vi "FanPressure2.vi"() -> ()   [LabVIEW 2024]
uses:
  <vilib>/drjdpowell/SQLite Library/SQL Connection/Connection.lvclass
  <vilib>/Instr/_visa.llb/VISA Find Search Mode.ctl
  <vilib>/drjdpowell/SQLite Library/SQL Connection/Open (path).vi
  <vilib>/Analysis/baseanly.llb/Mean (DBL).vi
  <vilib>/drjdpowell/SQLite Library/SQL Connection/Open (string).vi
  <vilib>/Instr/_visa.llb/VISA Configure Serial Port (Instr).vi
  <vilib>/drjdpowell/SQLite Library/SQL Connection/Execute SQL (No results).vi
  <vilib>/AdvancedString/Path To Command Line String.vi
  <vilib>/Analysis/NI_AALBase.lvlib
  <vilib>/drjdpowell/SQLite Library/SQLite.lvlib
panel:
  out "Array":string[](array[string])
  in  "Pause":bool
  out "DC Power":bool
  in  "Message":string
  out "Receive Type":T1
  out "user event out":refnum<user-event>
  out "Table Name":string
  out "Table Created":bool
  out "time string":string
  out "date string":string
  out "SQLite Connection":refnum<class "Connection.lvclass">
  in  "View Data":bool
  in  "Reset Plot":bool
  in  "Write To Database":bool
  in  "Interval Time":u32=200
  out "Fan Speed":i32
  out "Fan Shunt Voltage":u16
  out "Fan Power":sgl
  out "Fan current":sgl
  out "Fan Voltage":sgl
  in  "Speed Control":enum32{"Values", "Paramters"}(tab)
  in  "Control Mode":enum32{"Auto", "Manual"}(radio)=enum."Manual"
  in  "Speed Setup":u16=2000 min=10 max=36 step=1
  in  "Output":sgl(knob) min=0 max=12 step=0.1 scale=0.0..12.0 scale format="%.1f"
  in  "Min Voltage":u32 max=12 step=1
  in  "Max Voltage":u32=12 min=12 max=36
  in  "Parameter Read Button":bool
  in  "Parameter Write Button":bool
  in  "Fan Speed At Full Output":u32
  in  "Fan Speed At 50% Output":u32
  in  "KD":sgl
  in  "KI":sgl=0.0002
  in  "KP":sgl=0.008
  in  "Write Data":bool
  in  "Start Button":bool
  out "MCU":bool
  out "Serial Port":refnum<visa-resource-name>
  in  "stop":bool
  in  "Tab Control":enum32{"Readings", "Raw Data"}(tab)
  out "Waveform Chart 2":dbl[][](graph)
  out "Waveform Chart":sgl[][](graph)
  out "data":dynamicdata(graph) caption="Raw Data"
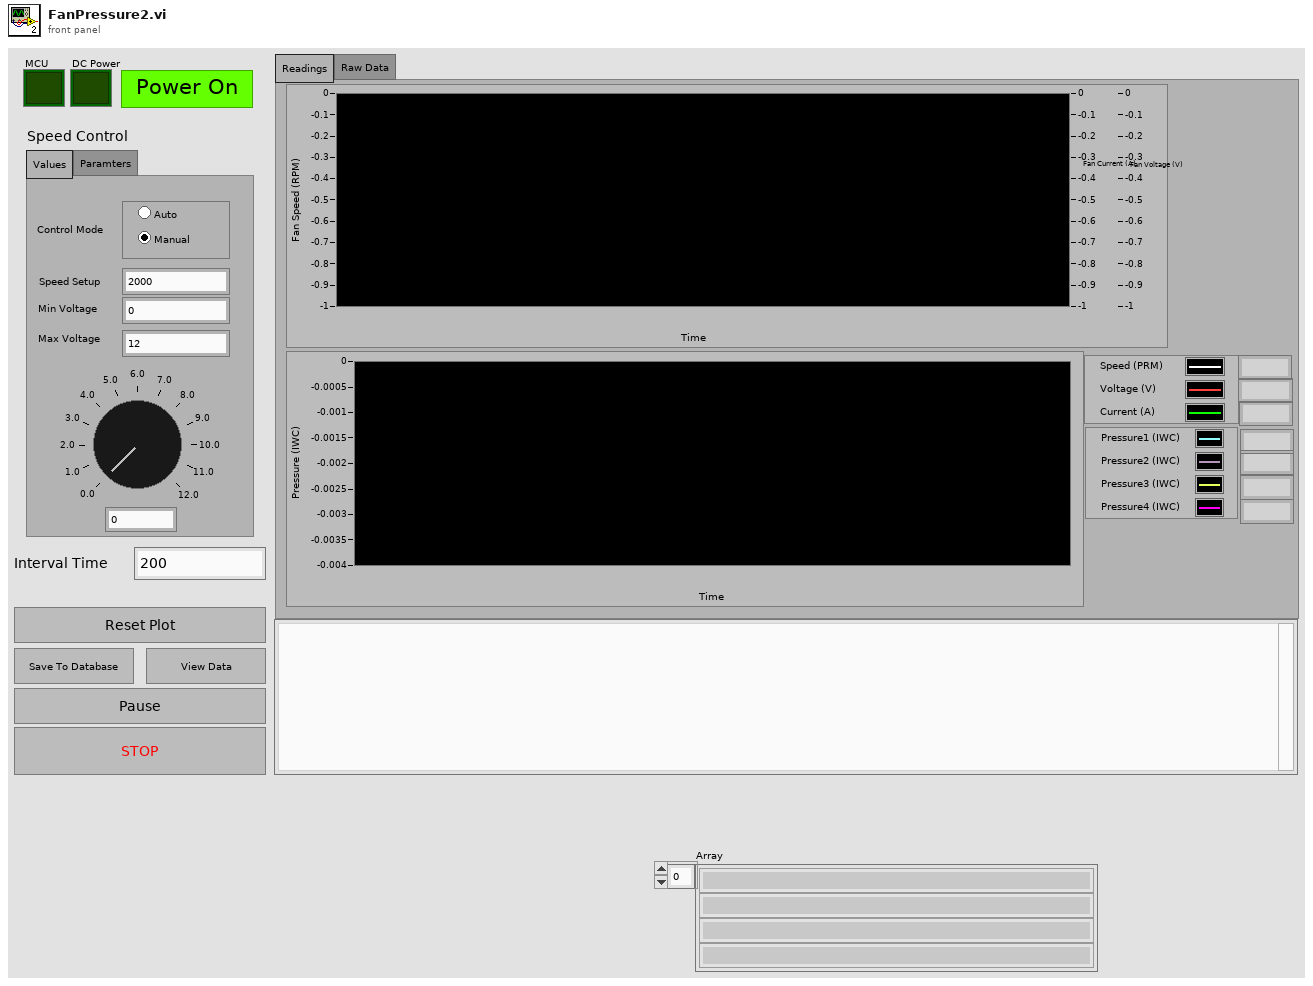
[diagram p1: front panel]
types:
  T1 = cluster{u8, u8, u8, u8, u16, u16, i16, i16, i16, i16, u16, u16, u16, u16, u16, u16, sgl, sgl, sgl, u32, u32, u8, u8, u8, u8}
  T2 = enum16{"New or existing", "Existing", "Read only"}
  T3 = enum8{"Enabled", "Disabled", "Disabled and Grayed Out"}
  T4 = enum32{"Invalid", "Standard", "Closed", "Hidden", "Minimized", "Maximized"}
  T5 = cluster{u32, "Fan current":sgl, "Fan current":sgl, "Fan current":sgl, "Fan Power":sgl, sgl, sgl, sgl, sgl, sgl, "Output":sgl, "Output":sgl}
  T6 = enum16{"big-endian, network order", "native, host order", "little-endian"}
  T7 = typedef "VISA Find Search Mode.ctl" = u32
  T8 = cluster{"y":u8, "y":u8, "y":u8, u8, u16, "Speed Setup":u16, u16, u16, "y":u8, "y":u8, "y":u8, "y":u8}
  T9 = cluster{"y":u8, "y":u8, "y":u8, "y":u8, "KP":sgl, "KI":sgl, "KD":sgl, "Fan Speed At 50% Output":u32, "Fan Speed At Full Output":u32, "y":u8, "y":u8, "y":u8, "y":u8}
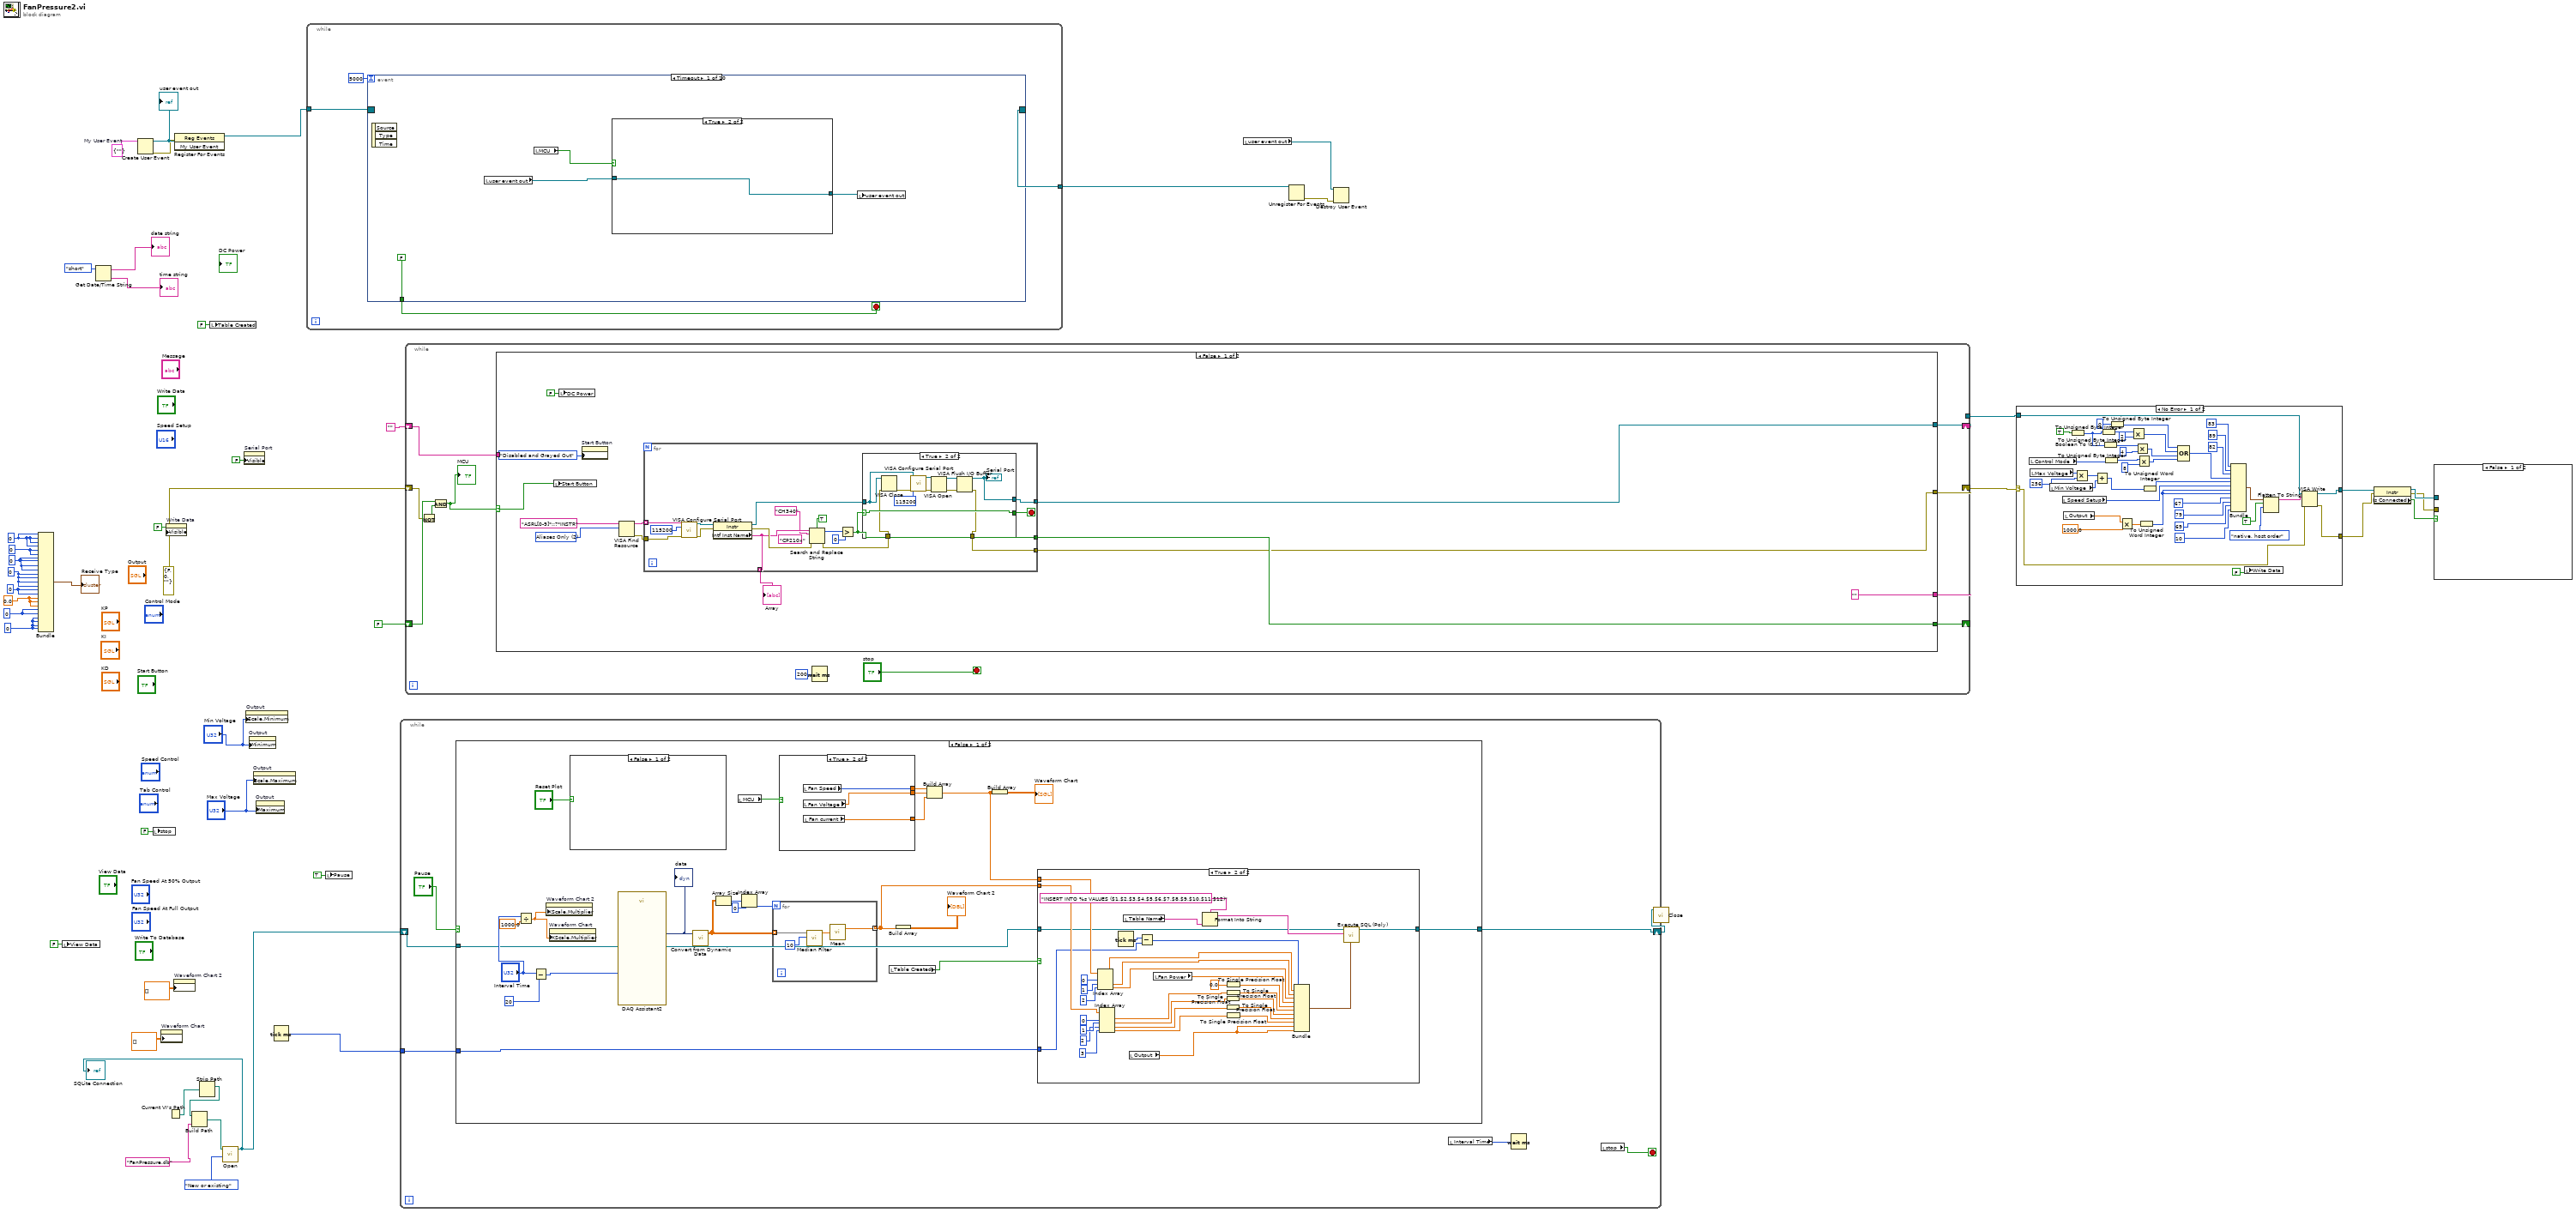
[diagram p0: block diagram]
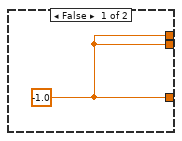
[diagram p3: hidden frame]
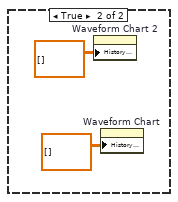
[diagram p4: hidden frame]
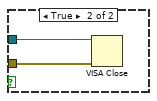
[diagram p6: hidden frame]
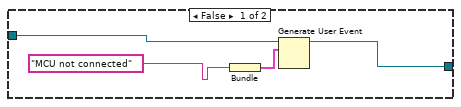
[diagram p8: hidden frame]
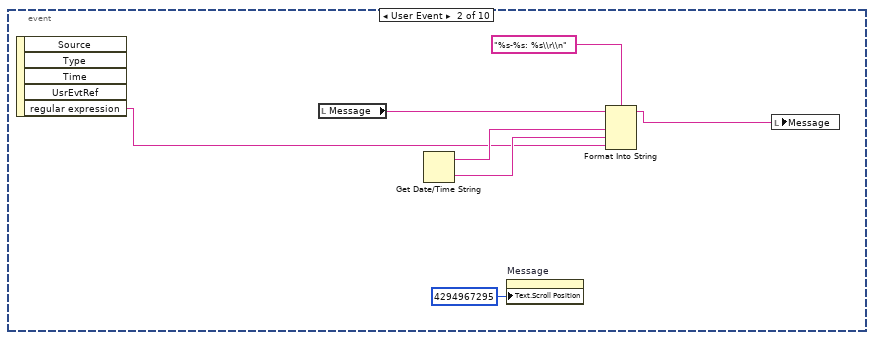
[diagram p9: hidden frame]
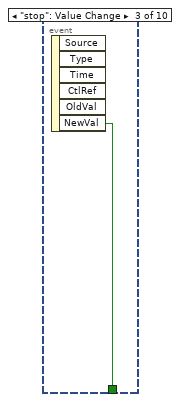
[diagram p10: hidden frame]
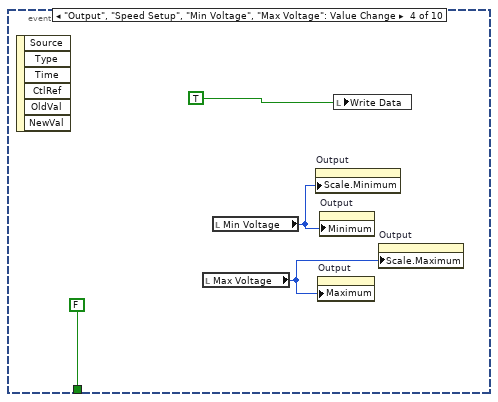
[diagram p11: hidden frame]
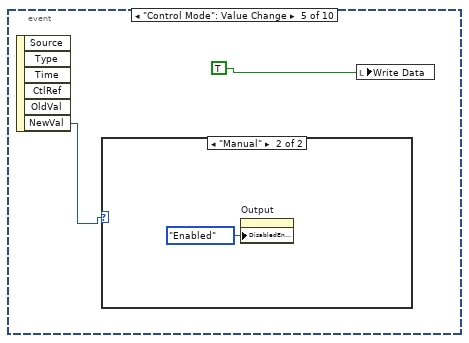
[diagram p12: hidden frame]
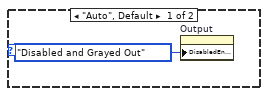
[diagram p13: hidden frame]
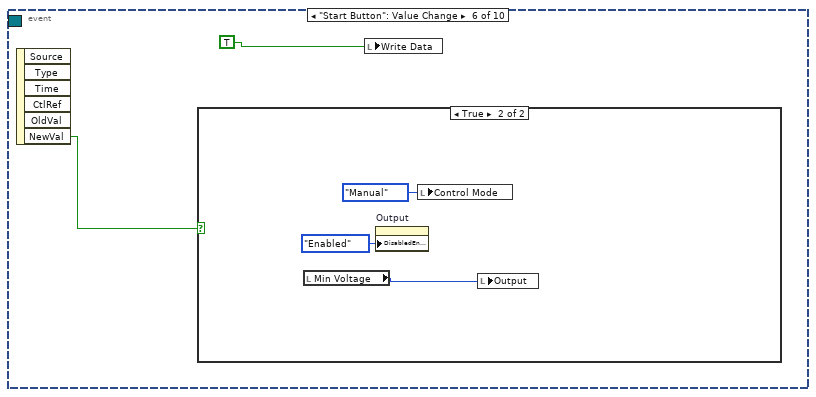
[diagram p14: hidden frame]
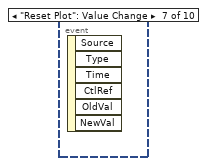
[diagram p16: hidden frame]
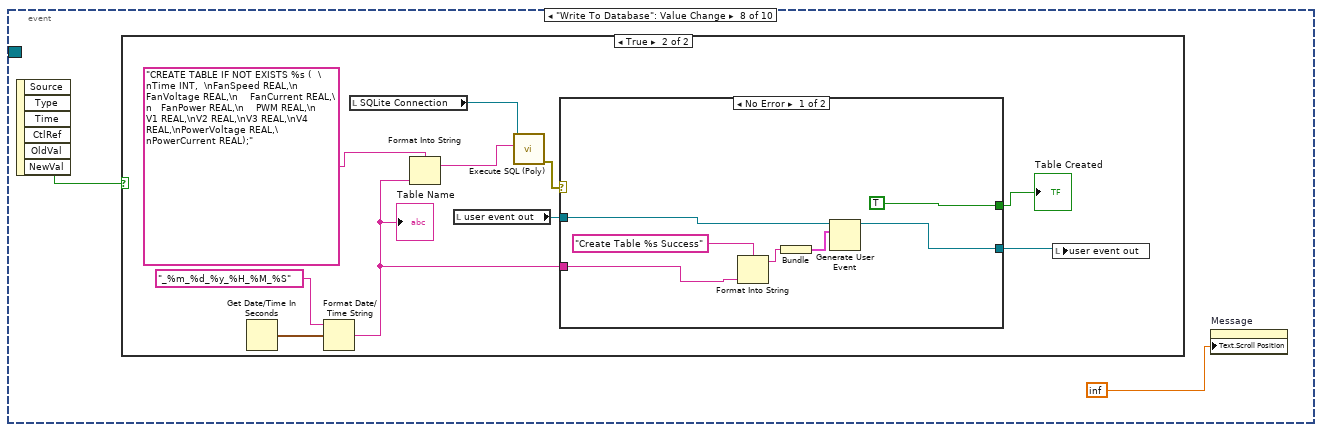
[diagram p17: hidden frame]
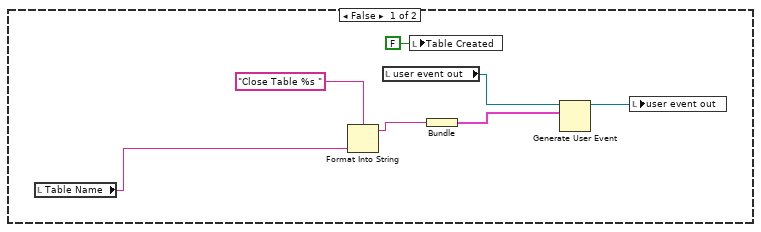
[diagram p18: hidden frame]
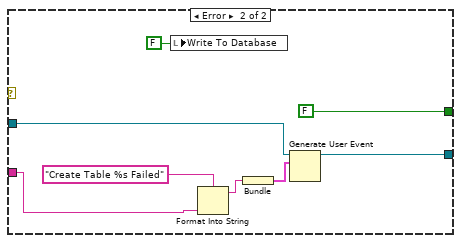
[diagram p19: hidden frame]
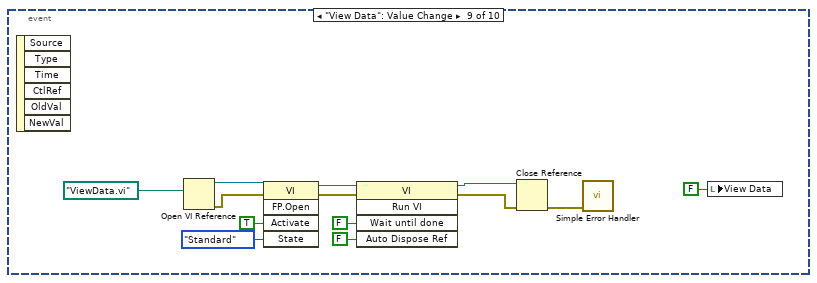
[diagram p20: hidden frame]
diagram:
  w3 = u32 0
  w4 = sgl 0.0
  w23 = cluster{"regular expression":string} {"regular expression"=""}  # My User Event
  w39 = u16 0
  w5 = u8 0
  w41 = i16 0
  w40 = u16 0
  w42 = u16 0
  w43 = u8 0
  n1 = Bundle(w43, w43, w43, w43, w42, w42, w41, w41, w41, w41, w39, w39, w39, w39, w40, w40, w4, w4, w4, w3, w3, w5, w5, w5, w5) -> (→"Receive Type":T1)  [unwired: 1 in]
  n2 = local write "View Data"(FALSE ("View Data")) -> ()
  n3 = Get Date/Time String(date format (0)=enum16{"short", "long", "abbreviated"}."short") -> (date string=→"date string":string, time string=→"time string":string)  [unwired: 2 in]
  n4 = Create User Event(user event datatype=w23) -> (user event=w22:refnum<user-event>, error out=w20:errorcluster)  [unwired: 1 in]
  "user event out" <- w22
  n5 = local write "stop"(FALSE ("stop")) -> ()
  n6 = property on="Waveform Chart" class="WFChart (strict)"("History Data"=dbl[][] []) -> ()  [unwired: 2 in, 2 out]
  n7 = property on="Write Data" class="Bool (strict)"("Visible"=FALSE) -> ()  [unwired: 2 in, 2 out]
  n8 = Current VI's Path() -> (path=w14:path)
  n9 = property on="Waveform Chart 2" class="WFChart (strict)"("History Data"=dbl[][] []) -> ()  [unwired: 2 in, 2 out]
  n10 = register-events(error in=w20, w22) -> (reference out=w21:refnum<event-registration>)  [unwired: 1 in, 1 out]
  n11 = Strip Path(path=w14) -> (stripped path=w13:path)  [unwired: 1 out]
  n12 = Build Path(base path=w13, name or relative path="FanPressure.db" ("db file")) -> (appended path=w15:path)
  n13 = local write "Table Created"(FALSE ("Table Created")) -> ()
  n14 = call-poly <vilib>:"Open.vi"("File Option"=T2."New or existing", "db file"=w15) -> ("SQLite Connection"=w12:refnum<class "Connection.lvclass">)  [unwired: 8 in, 1 out]
  "SQLite Connection" <- w12
  n15 = property on="Serial Port" class="VISAName"("Visible"=FALSE) -> ()  [unwired: 2 in, 2 out]
  n16 = property on="Output" class="Knob (strict)"("Scale.Minimum"="Min Voltage") -> ()  [unwired: 2 in, 2 out]
  n17 = property on="Output" class="Knob (strict)"("Minimum"="Min Voltage") -> ()  [unwired: 2 in, 2 out]
  n18 = property on="Output" class="Knob (strict)"("Scale.Maximum"="Max Voltage") -> ()  [unwired: 2 in, 2 out]
  n19 = property on="Output" class="Knob (strict)"("Maximum"="Max Voltage") -> ()  [unwired: 2 in, 2 out]
  n20 = Tick Count (ms)() -> (millisecond timer value=w9:u32)
  n21 = while {
    tunnel: w21 -> [w50]
    tunnel: [w49] -> w19
    stop <- w51 stop-if-true
    n22 = event shown="[0] Timeout" {
      selector: w50 -> [_ _ _ _ _ _ _ _ _ _]
      dyn-events: [_ _ _ _ _ _ _ _ _ _] -> w49
      timeout: 5000 -> [_ _ _ _ _ _ _ _ _ _]
      tunnel: [FALSE ("NewVal") _ w68 FALSE ("NewVal") _ _ _ _ _ _] -> w51
      event Timeout {
        n23 = event-data() -> ()  [unwired: 1 in, 3 out]
        n24 = local read "user event out"() -> (w54:refnum<user-event>)
        n25 = local read "MCU"() -> (w52:bool)
        n26 = case shown="True" w52 {
          tunnel: w54 -> [w57 w60]
          tunnel: [w58 w60] -> w53
          frame False {
            n27 = Bundle("format string"="MCU not connected") -> (w59:cluster{"format string":string})  [unwired: 1 in]
            n28 = Generate User Event(user event=w57, event data cluster=w59) -> (user event out=w58:refnum<user-event>)  [unwired: 2 in, 1 out]
          }
          frame True {
          }
        }
        n29 = local write "user event out"(w53) -> ()
      }
      event User Event {
        n30 = event-data() -> ("regular expression"=w62:string)  [unwired: 1 in, 4 out]
        n31 = local read "Message"() -> (w67:string)
        n32 = Get Date/Time String() -> (date string=w66:string, time string=w65:string)  [unwired: 3 in]
        n33 = property on="Message" class="Str"("Text.Scroll Position"=u32 4294967295) -> ()  [unwired: 2 in, 2 out]
        n34 = Format Into String(format string="%s-%s: %s\\r\\n", initial string=w67, w66, w65, w62) -> (resulting string=w64:string)  [unwired: 1 in, 1 out]
        n35 = local write "Message"(w64) -> ()
      }
      event "stop": Value Change {
        n36 = event-data() -> ("NewVal"=w68:bool)  [unwired: 1 in, 5 out]
      }
      event "Output", "Speed Setup", "Min Voltage", "Max Voltage": Value Change {
        n37 = event-data() -> ()  [unwired: 1 in, 6 out]
        n38 = local read "Max Voltage"() -> (w69:u32)
        n39 = local read "Min Voltage"() -> (w70:u32)
        n40 = property on="Output" class="Knob (strict)"("Scale.Minimum"=w70) -> ()  [unwired: 2 in, 2 out]
        n41 = property on="Output" class="Knob (strict)"("Maximum"=w69) -> ()  [unwired: 2 in, 2 out]
        n42 = property on="Output" class="Knob (strict)"("Minimum"=w70) -> ()  [unwired: 2 in, 2 out]
        n43 = local write "Write Data"(TRUE ("Write Data")) -> ()
        n44 = property on="Output" class="Knob (strict)"("Scale.Maximum"=w69) -> ()  [unwired: 2 in, 2 out]
      }
      event "Control Mode": Value Change {
        n45 = event-data() -> ("NewVal"=w73:enum32{"Auto", "Manual"})  [unwired: 1 in, 5 out]
        n46 = case shown="\"Manual\"" w73 {
          frame "Auto", Default {
            n47 = property on="Output" class="Knob (strict)"("DisabledEnum"=T3."Disabled and Grayed Out" ("Disabled")) -> ()  [unwired: 2 in, 2 out]
          }
          frame "Manual" {
            n48 = property on="Output" class="Knob (strict)"("DisabledEnum"=T3."Enabled" ("Disabled")) -> ()  [unwired: 2 in, 2 out]
          }
        }
        n49 = local write "Write Data"(TRUE ("Write Data")) -> ()
      }
      event "Start Button": Value Change {
        n50 = event-data() -> ("NewVal"=w77:bool)  [unwired: 1 in, 5 out]
        n51 = case shown="True" w77 {
          frame False {
          }
          frame True {
            n52 = local read "Min Voltage"() -> (w80:u32)
            n53 = property on="Output" class="Knob (strict)"("DisabledEnum"=T3."Enabled" ("Disabled")) -> ()  [unwired: 2 in, 2 out]
            n54 = local write "Control Mode"(enum32{"Auto", "Manual"}."Manual" ("Control Mode")) -> ()
            n55 = local write "Output"(w80) -> ()
          }
        }
        n56 = local write "Write Data"(TRUE ("Write Data")) -> ()
      }
      event "Reset Plot": Value Change {
        n57 = event-data() -> ()  [unwired: 1 in, 6 out]
      }
      event "Write To Database": Value Change {
        n58 = event-data() -> ("NewVal"=w83:bool)  [unwired: 1 in, 5 out]
        n59 = case shown="True" w83 {
          frame False {
            n60 = local read "Table Name"() -> (w89:string)
            n61 = Format Into String(format string="Close Table %s ", w89) -> (resulting string=w86:string)  [unwired: 2 in, 1 out]
            n62 = local read "user event out"() -> (w87:refnum<user-event>)
            n63 = local write "Table Created"(FALSE ("Table Created")) -> ()
            n64 = Bundle(w86) -> (w85:cluster{string})  [unwired: 1 in]
            n65 = Generate User Event(user event=w87, event data cluster=w85) -> (user event out=w84:refnum<user-event>)  [unwired: 2 in, 1 out]
            n66 = local write "user event out"(w84) -> ()
          }
          frame True {
            n67 = Get Date/Time In Seconds() -> (seconds since 1Jan1904=w99:timestamp)
            n68 = Format Date/Time String(time format string (%c)="_%m_%d_%y_%H_%M_%S", seconds (now)=w99) -> (date/time string=w91:string)  [unwired: 1 in]
            "Table Name" <- w91
            n69 = local read "SQLite Connection"() -> (w100:refnum<class "Connection.lvclass">)
            n70 = Format Into String(format string="CREATE TABLE IF NOT EXISTS %s (  \nTime INT,  \nFanSpeed REAL,\n    FanVoltage REAL,\n    FanCurrent REAL,\n   FanPower REAL,\n    PWM REAL,\n    V1 REAL,\nV2 REAL,\nV3 REAL,\nV4 REAL,\nPowerVoltage REAL,\nPowerCurrent REAL);" ("SQL"), w91) -> (resulting string=w96:string)  [unwired: 2 in, 1 out]
            n71 = local read "user event out"() -> (w93:refnum<user-event>)
            n72 = call-poly <vilib>:"Execute SQL (Poly).vi"("SQL"=w96, "SQLite Connection in"=w100) -> ("error out"=w95:errorcluster)  [unwired: 8 in, 1 out]
            n73 = case shown="No Error" w95 {
              tunnel: [TRUE ("Table Created") FALSE ("Table Created")] -> w94
              tunnel: w93 -> [w101 w110]
              tunnel: [w102 w109] -> w92
              tunnel: w91 -> [w103 w108]
              frame No Error {
                n74 = Format Into String(format string="Create Table %s Success", w103) -> (resulting string=w106:string)  [unwired: 2 in, 1 out]
                n75 = Bundle(w106) -> (w105:cluster{string})  [unwired: 1 in]
                n76 = Generate User Event(user event=w101, event data cluster=w105) -> (user event out=w102:refnum<user-event>)  [unwired: 2 in, 1 out]
              }
              frame Error {
                n77 = local write "Write To Database"(FALSE ("Write To Database")) -> ()
                n78 = Format Into String(format string="Create Table %s Failed", w108) -> (resulting string=w113:string)  [unwired: 2 in, 1 out]
                n79 = Bundle(w113) -> (w112:cluster{string})  [unwired: 1 in]
                n80 = Generate User Event(user event=w110, event data cluster=w112) -> (user event out=w109:refnum<user-event>)  [unwired: 2 in, 1 out]
              }
            }
            "Table Created" <- w94
            n81 = local write "user event out"(w92) -> ()
          }
        }
        n82 = property on="Message" class="Str"("Text.Scroll Position"=inf) -> ()  [unwired: 2 in, 2 out]
      }
      event "View Data": Value Change {
        n83 = event-data() -> ()  [unwired: 1 in, 6 out]
        n84 = Open VI Reference(vi path=path "ViewData.vi") -> (vi reference=w126:refnum<vi>, error out=w119:errorcluster)  [unwired: 5 in]
        n85 = invoke class="VI" method="FP.Open"(reference=w126, error in=w119, "Activate"=TRUE ("Activate?"), "State"=T4."Standard") -> (reference out=w123:refnum<vi>, error out=w122:errorcluster)  [unwired: 1 in, 3 out]
        n86 = invoke class="VI" method="Run VI"(reference=w123, error in=w122, "Wait until done"=FALSE ("Wait Until Done"), "Auto Dispose Ref"=FALSE ("Auto Dispose Reference")) -> (reference out=w118:refnum<vi>, error out=w117:errorcluster)  [unwired: 1 in, 3 out]
        n87 = Close Reference(reference=w118, error in (no error)=w117) -> (error out=w116:errorcluster)
        n88 = call <vilib>:"Simple Error Handler.vi"("error in (no error)"=w116) -> ()  [unwired: 4 in, 5 out]
        n89 = local write "View Data"(FALSE ("View Data")) -> ()
      }
      event "Message": Value Change {
        n90 = event-data() -> ()  [unwired: 1 in, 6 out]
      }
    }
  }
  n91 = local write "Pause"(TRUE ("Pause")) -> ()
  n92 = while {
    shift-right: [w132] -> w11
    shift-left: w12 -> [w131]
    tunnel: w9 -> [w130]
    stop <- w134 stop-if-true
    n93 = case shown="False" "Pause" {
      tunnel: [w137 w202] -> w132
      tunnel: w131 -> [w136 w202]
      tunnel: w130 -> [w135 _]
      frame False {
        n94 = Divide(x="Interval Time", y=1000.0) -> (x/y=w146:dbl)
        n95 = Subtract(x="Interval Time", y=u32 20) -> (x-y=w155:u32)
        n96 = property on="Waveform Chart 2" class="WFChart (strict)"("XScale.Multiplier"=w146) -> ()  [unwired: 2 in, 2 out]
        n97 = property on="Waveform Chart" class="WFChart (strict)"("XScale.Multiplier"=w146) -> ()  [unwired: 2 in, 2 out]
        n98 = case shown="False" "Reset Plot" {
          frame False {
          }
          frame True {
            n99 = property on="Waveform Chart 2" class="WFChart (strict)"("History Data"=dbl[][] []) -> ()  [unwired: 2 in, 2 out]
            n100 = property on="Waveform Chart" class="WFChart (strict)"("History Data"=dbl[][] []) -> ()  [unwired: 2 in, 2 out]
          }
        }
        n101 = call "DAQ Assistant2"("number of samples"=w155) -> ("data"=w157:dynamicdata)  [unwired: 16 in, 2 out]
        "data" <- w157
        n102 = call "Convert from Dynamic Data"("Dynamic Data Type"=w157) -> ("Array"=w154:dbl[][])  [unwired: 3 in]
        n103 = Array Size(array=w154) -> (size(s)=w153:i32[])
        n104 = local read "MCU"() -> (w145:bool)
        n105 = Index Array(array=w153, index=0) -> (element=w151:i32)
        n106 = for {
          N: w151 -> [_]
          tunnel: w154 -> [w201] mode=indexing
          tunnel: [w198] -> w140 mode=indexing
          n107 = call <vilib>:"Median Filter.vi"("left rank"=10, "X"=w201) -> ("Filtered X"=w199:dbl[])  [unwired: 8 in, 1 out]
          n108 = call-poly <vilib>:"Mean.vi"("X"=w199) -> ("mean"=w198:dbl)  [unwired: 1 out]
        }
        n109 = case shown="True" w145 {
          tunnel: [w192 w195] -> w144
          tunnel: [w192 w194] -> w143
          tunnel: [w192 w193] -> w142
          frame False {
            w192 = sgl -1.0 ("Fan current")
          }
          frame True {
            n110 = local read "Fan Speed"() -> (w193:i32)
            n111 = local read "Fan Voltage"() -> (w194:sgl)
            n112 = local read "Fan current"() -> (w195:sgl)
          }
        }
        n113 = local read "Table Created"() -> (w138:bool)
        n114 = Build Array(w140) -> (→"Waveform Chart 2":dbl[][])
        n115 = Build Array(w142, w143, w144) -> (w139:sgl[])
        n116 = Build Array(w139) -> (→"Waveform Chart":sgl[][])
        n117 = case shown="True" w138 {
          tunnel: w140 -> [_ w187]
          tunnel: w139 -> [_ w191]
          tunnel: w136 -> [w158 w174]
          tunnel: [w158 w173] -> w137
          tunnel: w135 -> [_ w162]
          frame False {
          }
          frame True {
            n118 = Index Array(array=w191, index #1=0 ("index"), index #2=1 ("index"), index #3=2 ("index")) -> (element #1=w182:sgl, element #2=w181:sgl, element #3=w180:sgl)
            n119 = Index Array(array=w187, index #1=0 ("index"), index #2=1 ("index"), index #3=2 ("index"), index #4=3 ("index")) -> (element #1=w166:dbl, element #2=w168:dbl, element #3=w170:dbl, element #4=w172:dbl)
            n120 = Tick Count (ms)() -> (millisecond timer value=w163:u32)
            n121 = local read "Table Name"() -> (w176:string)
            n122 = local read "Output"() -> (w159:sgl)
            n123 = Subtract(x=w163, y=w162) -> (x-y=w161:u32)
            n124 = local read "Fan Power"() -> (w179:sgl)
            n125 = Format Into String(format string="INSERT INTO %s VALUES ($1,$2,$3,$4,$5,$6,$7,$8,$9,$10,$11,$12)" ("SQL"), w176) -> (resulting string=w175:string)  [unwired: 2 in, 1 out]
            n126 = To Single Precision Float(number=w168) -> (single precision float=w167:sgl)
            n127 = To Single Precision Float(number=w170) -> (single precision float=w169:sgl)
            n128 = To Single Precision Float(number=sgl 0.0) -> (single precision float=w164:sgl)
            n129 = To Single Precision Float(number=w166) -> (single precision float=w165:sgl)
            n130 = To Single Precision Float(number=w172) -> (single precision float=w171:sgl)
            n131 = Bundle(w161, "Fan current"=w182, "Fan current"=w181, "Fan current"=w180, "Fan Power"=w179, w164, w165, w167, w169, w171, "Output"=w159, "Output"=w159) -> (w178:T5)  [unwired: 1 in]
            n132 = call-poly <vilib>:"Execute SQL (Poly).vi"("Parameter(s)"=w178, "SQL"=w175, "SQLite Connection in"=w174) -> ("SQLite Connection"=w173:refnum<class "Connection.lvclass">)  [unwired: 7 in, 1 out]
          }
        }
      }
      frame True {
      }
    }
    n133 = local read "Interval Time"() -> (w133:u32)
    n134 = Wait (ms)(milliseconds to wait=w133) -> ()  [unwired: 1 out]
    n135 = local read "stop"() -> (w134:bool)
  }
  n136 = while {
    shift-right: [w212] -> _
    shift-left: FALSE -> [w210]
    shift-right: [w211] -> w36
    shift-left: errorcluster {"status"=FALSE, "code"=0, "source"=""} ("error in (no error)") -> [w206]
    tunnel: [w208] -> w37
    shift-right: [w205] -> _
    shift-left: "" -> [w204]
    stop <- "stop" stop-if-true
    n137 = Not(x=w206) -> (.not. x?=w209:bool)
    n138 = And(x=w210, y=w209) -> (x .and. y?=w203:bool)
    "MCU" <- w203
    n139 = case shown="False" w203 {
      selector: w203 -> [w217 w271]
      tunnel: [w221 w271] -> w212
      tunnel: [w220 w264] -> w211
      tunnel: [w219 w266] -> w208
      tunnel: w204 -> [_ w276]
      tunnel: ["" w260] -> w205
      frame False {
        w224 = T7 2 items=["Canonical Names Only"=0, "Aliases Only"=2, "Include Matching Aliases"=3, "Include All Aliases"=4] ("Search Mode")
        n140 = local write "Start Button"(w217) -> ()
        n141 = local write "DC Power"(FALSE ("DC Power")) -> ()
        n142 = property on="Start Button" class="Bool (strict)"("DisabledEnum"=T3."Disabled and Grayed Out" ("Disabled")) -> ()  [unwired: 2 in, 2 out]
        n143 = VISA Find Resource(10:w224, 11:"ASRL[0-9]*::?*INSTR" ("expression (\"?*\")")) -> (0:w222:errorcluster, 3:w223:string[])  [unwired: 1 in, 1 out]
        n144 = for {
          tunnel: w223 -> [w232] mode=indexing
          tunnel: w222 -> [w242]
          tunnel: [w236] -> w221
          tunnel: [w229] -> w220
          tunnel: [w228] -> w219
          tunnel: [w227] -> w214 mode=indexing
          stop <- w235 stop-if-true
          (unwired) "CP210x" ("search string")
          n145 = call-poly "VISA Configure Serial Port"("VISA resource name"=w232, "baud rate (9600)"=u32 115200, "error in (no error)"=w242) -> ("VISA resource name out"=w231:refnum<visa-resource-name>, "error out"=w241:errorcluster)  [unwired: 11 in]
          n146 = property class="Instr"(reference=w231, error in=w241) -> (reference out=w234:refnum<visa-resource-name>, error out=w240:errorcluster, "Intf Inst Name"=w227:string)
          n147 = Search and Replace String(case sensitive?=TRUE ("ignore case? (F)"), input string=w227, search string="CH340", error in=w240) -> (number of replacements=w238:i32, error out=w230:errorcluster)  [unwired: 4 in, 2 out]
          n148 = Greater?(x=w238, y=0) -> (0:w236:bool)
          n149 = case shown="True" w236 {
            selector: w236 -> [w246 w257]
            tunnel: [w246 w257] -> w235
            tunnel: w234 -> [w243 w255]
            tunnel: w230 -> [w245 w256]
            tunnel: [w244 w249] -> w229
            tunnel: [w243 w251] -> w228
            frame False {
              n150 = VISA Close(VISA resource name=w243, error in (no error)=w245) -> (error out=w244:errorcluster)
            }
            frame True {
              n151 = VISA Close(VISA resource name=w255, error in (no error)=w256) -> (error out=w248:errorcluster)
              n152 = call-poly "VISA Configure Serial Port"("VISA resource name"=w255, "baud rate (9600)"=u32 115200, "error in (no error)"=w248) -> ("VISA resource name out"=w253:refnum<visa-resource-name>, "error out"=w247:errorcluster)  [unwired: 11 in]
              n153 = VISA Open(error in (no error)=w247, VISA resource name=w253) -> (VISA resource name=w252:refnum<visa-resource-name>, error out=w250:errorcluster)  [unwired: 3 in]
              n154 = VISA Flush I/O Buffer(VISA resource name=w252, error in (no error)=w250) -> (VISA resource name out=w251:refnum<visa-resource-name>, error out=w249:errorcluster)  [unwired: 1 in]
              "Serial Port" <- w251
            }
          }
        }
        "Array" <- w214
      }
      frame True {
        n155 = local read "Serial Port"() -> (w281:refnum<visa-resource-name>)
        n156 = property class="Instr"(reference=w281) -> (reference out=w279:refnum<visa-resource-name>, error out=w278:errorcluster, "Serial Settings:Number of Bytes at Serial Port"=w280:u32)  [unwired: 1 in]
        n157 = property on="Start Button" class="Bool (strict)"("DisabledEnum"=T3."Enabled" ("Disabled")) -> ()  [unwired: 2 in, 2 out]
        n158 = VISA Read(VISA resource name=w279, byte count=w280, error in (no error)=w278) -> (VISA resource name out=w272:refnum<visa-resource-name>, read buffer=w277:string, error out=w268:errorcluster)  [unwired: 1 out]
        n159 = Concatenate Strings(w276, w277) -> (w259:string)
        n160 = Match Pattern(string=w259, regular expression="SU.*COE\\n") -> (match substring=w261:string, after substring=w258:string)  [unwired: 1 in, 2 out]
        n161 = String Length(string=w261) -> (length=w274:i32)
        n162 = Greater?(x=w274, y=0) -> (0:w262:bool)
        n163 = case shown="True" w262 {
          tunnel: [w282 w283] -> w260
          tunnel: w258 -> [_ w283]
          tunnel: w259 -> [w282 _]
          frame False {
          }
          frame True {
          }
        }
        n164 = case shown="True" w262 {
          tunnel: w261 -> [_ w388]
          frame False {
          }
          frame True {
            w354 = u8 2 ("y")
            n165 = local read "Receive Type"() -> (w365:T1)
            n166 = Unflatten From String(type=w365, binary string=w388, byte order (0:big-endian, network order)=T6."native, host order") -> (value=w386:T1)  [unwired: 2 in, 2 out]
            n167 = Unbundle(w386) -> (w356:u8, w385:u16, w383:u16, w380:u16, w376:u16, w374:u16, →"Fan Shunt Voltage":u16, w370:u16, w368:u16, w363:sgl, w362:sgl, w361:sgl, w360:u32, w359:u32)  [unwired: 11 out]
            n168 = case shown="True" "Parameter Read Button" {
              tunnel: w363 -> [_ w398]
              tunnel: w362 -> [_ w397]
              tunnel: w361 -> [_ w396]
              tunnel: w360 -> [_ w395]
              tunnel: w359 -> [_ w394]
              frame False {
              }
              frame True {
                n169 = local write "Fan Speed At Full Output"(w394) -> ()
                n170 = local write "Fan Speed At 50% Output"(w395) -> ()
                n171 = local write "KP"(w398) -> ()
                n172 = local write "KI"(w397) -> ()
                n173 = local write "KD"(w396) -> ()
              }
            }
            n174 = Quotient & Remainder(x=w356, y=w354) -> (x-y*floor(x/y)=w357:u8, floor(x/y)=w355:u8)
            n175 = case shown="0, Default" w357 {
              frame 0, Default {
                n176 = local write "DC Power"(FALSE ("DC Power")) -> ()
                n177 = local write "Control Mode"(enum32{"Auto", "Manual"}."Manual" ("Control Mode")) -> ()
              }
              frame 1 {
                n178 = local write "DC Power"(TRUE ("DC Power")) -> ()
              }
            }
            n179 = Quotient & Remainder(x=w355, y=w354) -> (x-y*floor(x/y)=w353:u8)  [unwired: 1 out]
            n180 = case shown="1" w353 {
              frame 0, Default {
              }
              frame 1 {
                n181 = local write "Write Data"(TRUE ("Write Data")) -> ()
              }
            }
            n182 = local read "Control Mode"() -> (w358:enum32{"Auto", "Manual"})
            n183 = Multiply(x=w380, y=0.00125) -> (x*y=→"Fan Voltage":dbl)
            n184 = Multiply(x=w385, y=0.1) -> (x*y=w366:dbl)
            n185 = Divide(x=w383, y=1000.0) -> ()  [unwired: 1 out]
            n186 = Multiply(x=w370, y=0.3) -> (x*y=→"Fan Speed":dbl)
            n187 = Multiply(x=w374, y=0.0025) -> (x*y=→"Fan Power":dbl)
            n188 = Multiply(x=w376, y=0.0001) -> (x*y=→"Fan current":dbl)
            n189 = Multiply(x=w368, y=0.001) -> ()  [unwired: 1 out]
            n190 = case shown="\"Auto\", Default" w358 {
              tunnel: w366 -> [w393 _]
              frame "Auto", Default {
                n191 = local write "Output"(w393) -> ()
              }
              frame "Manual" {
              }
            }
          }
        }
        n192 = local read "Write Data"() -> (w269:bool)
        n193 = case shown="True" w269 {
          tunnel: w272 -> [w308 w352]
          tunnel: [w308 w351] -> w267
          tunnel: w268 -> [w307 w350]
          tunnel: [w307 w349] -> w265
          frame False {
          }
          frame True {
            w315 = TRUE ("Boolean")
            n194 = local read "Max Voltage"() -> (w314:u32)
            n195 = local read "Control Mode"() -> (w316:enum32{"Auto", "Manual"})
            n196 = local read "Start Button"() -> (w345:bool)
            n197 = local read "Min Voltage"() -> (w311:u32)
            n198 = local read "Speed Setup"() -> (w329:u16)
            n199 = local read "Output"() -> (w327:sgl)
            n200 = Multiply(x=w314, y=u32 256) -> (x*y=w312:u32)
            n201 = Boolean To (0,1)(Boolean=w315) -> (0, 1=w344:i16)
            n202 = Boolean To (0,1)(Boolean=w345) -> (0, 1=w346:i16)
            n203 = Boolean To (0,1)(Boolean=w315) -> (0, 1=w347:i16)
            n204 = Add(x=w312, y=w311) -> (x+y=w310:u32)
            n205 = To Unsigned Byte Integer(number=w347) -> (unsigned 8bit integer=w339:u8)
            n206 = To Unsigned Byte Integer(number=w344) -> (unsigned 8bit integer=w336:u8)
            n207 = To Unsigned Byte Integer(number=w316) -> (unsigned 8bit integer=w335:u8)
            n208 = To Unsigned Byte Integer(number=w346) -> (unsigned 8bit integer=w343:u8)
            n209 = Multiply(x=w327, y=sgl 10.0) -> (x*y=w326:sgl)
            n210 = Multiply(x=w339, y=u8 2) -> (x*y=w337:u8)
            n211 = Multiply(x=w336, y=u8 4) -> (x*y=w331:u8)
            n212 = Multiply(x=w335, y=u8 8 ("x")) -> (x*y=w333:u8)
            n213 = To Unsigned Word Integer(number=w326) -> (unsigned 16bit integer=w325:u16)
            n214 = To Unsigned Word Integer(number=w310) -> (unsigned 16bit integer=w330:u16)
            n215 = Compound Arithmetic op=OR(w343, w337, w331, w333) -> (w342:u8)
            n216 = Bundle("y"=u8 83, "y"=u8 89, "y"=u8 82, w342, w330, "Speed Setup"=w329, w325, w325, "y"=u8 67, "y"=u8 79, "y"=u8 69, "y"=u8 10) -> (w317:T8)  [unwired: 1 in]
            n217 = local write "Write Data"(FALSE ("Write Data")) -> ()
            n218 = Flatten To String(anything=w317, prepend array or string size? (T)=TRUE, byte order (0:big-endian, network order)=T6."native, host order") -> (data string=w309:string)  [unwired: 1 in, 2 out]
            n219 = VISA Write(VISA resource name=w352, write buffer=w309, error in (no error)=w350) -> (VISA resource name out=w351:refnum<visa-resource-name>, error out=w349:errorcluster)  [unwired: 1 out]
          }
        }
        n220 = case shown="True" "Parameter Write Button" {
          tunnel: w267 -> [w285 w306]
          tunnel: [w285 w305] -> w266
          tunnel: w265 -> [w284 w302]
          tunnel: [w284 w303] -> w264
          frame False {
          }
          frame True {
            n221 = local read "Fan Speed At 50% Output"() -> (w294:u32)
            n222 = local read "Fan Speed At Full Output"() -> (w293:u32)
            n223 = local read "KD"() -> (w295:sgl)
            n224 = local read "KP"() -> (w297:sgl)
            n225 = local read "KI"() -> (w296:sgl)
            n226 = Bundle("y"=u8 67, "y"=u8 79, "y"=u8 69, "y"=u8 10, "KP"=w297, "KI"=w296, "KD"=w295, "Fan Speed At 50% Output"=w294, "Fan Speed At Full Output"=w293, "y"=u8 83, "y"=u8 89, "y"=u8 82, "y"=u8 10) -> (w288:T9)  [unwired: 1 in]
            n227 = Flatten To String(anything=w288, byte order (0:big-endian, network order)=T6."native, host order", error in (no error)=w302) -> (data string=w286:string, error out=w304:errorcluster)  [unwired: 1 in, 1 out]
            n228 = VISA Write(VISA resource name=w306, write buffer=w286, error in (no error)=w304) -> (VISA resource name out=w305:refnum<visa-resource-name>, error out=w303:errorcluster)  [unwired: 1 out]
          }
        }
      }
    }
    n229 = Wait (ms)(milliseconds to wait=u32 200) -> ()  [unwired: 1 out]
  }
  n230 = local read "user event out"() -> (w17:refnum<user-event>)
  n231 = Unregister For Events(event registration refnum=w19) -> (error out=w18:errorcluster)  [unwired: 1 in]
  n232 = Destroy User Event(user event=w17, error in=w18) -> ()  [unwired: 1 out]
  n233 = call-dynamic "Close.vi"("SQLite Connection in"=w11) -> ()  [unwired: 10 in, 1 out]
  n234 = case shown="No Error" w36 {
    selector: w36 -> [w407 w442]
    tunnel: [w440 w441] -> w34
    tunnel: [w439 w442] -> w33
    tunnel: w37 -> [w406 w441]
    frame No Error {
      n235 = local read "Control Mode"() -> (w408:enum32{"Auto", "Manual"})
      n236 = local read "Max Voltage"() -> (w403:u32)
      n237 = local read "Min Voltage"() -> (w401:u32)
      n238 = local read "Speed Setup"() -> (w423:u16)
      n239 = local read "Output"() -> (w420:sgl)
      n240 = Boolean To (0,1)(Boolean=TRUE) -> (0, 1=w404:i16)
      n241 = Multiply(x=w403, y=u32 256) -> (x*y=w402:u32)
      n242 = Add(x=w402, y=w401) -> (x+y=w399:u32)
      n243 = To Unsigned Byte Integer(number=w404) -> (unsigned 8bit integer=w433:u8)
      n244 = To Unsigned Byte Integer(number=w404) -> (unsigned 8bit integer=w430:u8)
      n245 = To Unsigned Byte Integer(number=w408) -> (unsigned 8bit integer=w429:u8)
      n246 = To Unsigned Byte Integer(number=u8 0) -> (unsigned 8bit integer=w437:u8)
      n247 = Multiply(x=w420, y=sgl 1000.0) -> (x*y=w419:sgl)
      n248 = Multiply(x=w433, y=u8 2) -> (x*y=w431:u8)
      n249 = Multiply(x=w430, y=u8 4) -> (x*y=w425:u8)
      n250 = Multiply(x=w429, y=u8 8 ("x")) -> (x*y=w427:u8)
      n251 = To Unsigned Word Integer(number=w419) -> (unsigned 16bit integer=w418:u16)
      n252 = To Unsigned Word Integer(number=w399) -> (unsigned 16bit integer=w424:u16)
      n253 = Compound Arithmetic op=OR(w437, w431, w425, w427) -> (w436:u8)
      n254 = Bundle("y"=u8 83, "y"=u8 89, "y"=u8 82, w436, w424, "Speed Setup"=w423, w418, w418, "y"=u8 67, "y"=u8 79, "y"=u8 69, "y"=u8 10) -> (w410:T8)  [unwired: 1 in]
      n255 = local write "Write Data"(FALSE ("Write Data")) -> ()
      n256 = Flatten To String(anything=w410, prepend array or string size? (T)=TRUE, byte order (0:big-endian, network order)=T6."native, host order") -> (data string=w409:string)  [unwired: 1 in, 2 out]
      n257 = VISA Write(VISA resource name=w406, write buffer=w409, error in (no error)=w407) -> (VISA resource name out=w440:refnum<visa-resource-name>, error out=w439:errorcluster)  [unwired: 1 out]
    }
    frame Error {
    }
  }
  n258 = property class="Instr"(reference=w34, error in=w33) -> (reference out=w31:refnum<visa-resource-name>, error out=w30:errorcluster, "Is Connected"=w32:bool)
  n259 = case shown="False" w32 {
    tunnel: w31 -> [_ w444]
    tunnel: w30 -> [_ w443]
    frame False {
    }
    frame True {
      n260 = VISA Close(VISA resource name=w444, error in (no error)=w443) -> ()  [unwired: 1 out]
    }
  }
